vi "Car Wash Controller.vi"(8 "error in (no error)":errorcluster, 9 "Module Routes":refnum<user-event>[](array[refnum]), 11 "Event Registration Refnum":refnum<event-registration>) -> (0 "error out":errorcluster)   [LabVIEW 2016]
doc: "Car wash controller main"
uses:
  Architecture/Message Queue/Message Cluster.ctl
  Controls/Controller Status.ctl
  Simulated Console/Controls/Button state.ctl
  Controls/Steps.ctl
  Controls/Stations.ctl
  Controls/Waiting States.ctl
  Architecture/Modules.ctl
  Simulated Console/Controls/Entry Display.ctl
  Architecture/Message Queue/Message Queue.lvlib
panel:
  in  "debug":bool
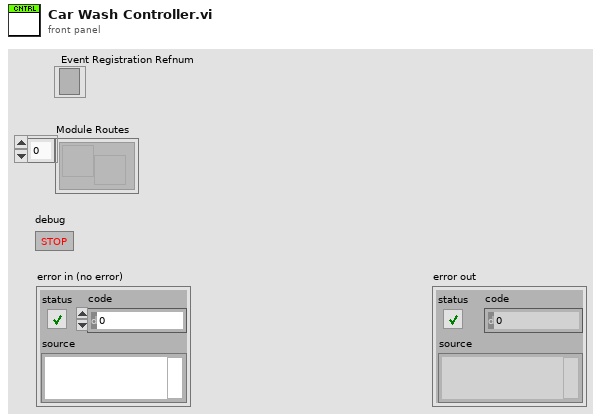
[diagram p1: front panel]
types:
  T1 = typedef "Controller Status.ctl" = cluster{"Module Routes":refnum<user-event>[], "Button States":T2[], "Current State":T3, "In Progress?":bool, "Out of Position?":bool, "Time Remaining":dbl, "Current Station":T4, "Waiting States":T5, "Chosen Cycles":cluster{"Under Body Wash":bool, "Bug Remover":bool, "Pre-Soak":bool, "High Pressure Wash (default)":bool, "Low Pressure Wax":bool, "Spot Free Rinse":bool, "Tire Shine Foam":bool, "Air Dry":bool}}
  T2 = typedef "Button state.ctl" = cluster{"Disabled State":enum8{"Enabled", "Disabled", "Disabled and Grayed Out"}, "State":bool}
  T3 = typedef "Steps.ctl" = enum16{"Under Body Wash", "Bug Remover", "Pre-Soak", "High Pressure Wash", "Low Pressure Wax", "Spot Free Rinse", "Tire Shine Foam", "Air Dry"}
  T4 = typedef "Stations.ctl" = enum16{"Entry", "Station 1", "Station 2", "Station 3", "Exit"}
  T5 = typedef "Waiting States.ctl" = enum16{"None", "for Start", "for Vehicle Position"}
  T6 = typedef "Entry Display.ctl" = cluster{"Text":string, "Color":u32}
  T7 = typedef "Modules.ctl" = enum16{"Database", "Car Wash Controller", "Console"}
  T8 = typedef "Error Severity.ctl" = enum16{"System Error", "Wash Error", "Minor"}
  T9 = cluster{"Under Body Wash":bool, "Bug Remover":bool, "Pre-Soak":bool, "High Pressure Wash (default)":bool, "Low Pressure Wax":bool, "Spot Free Rinse":bool, "Tire Shine Foam":bool, "Air Dry":bool}
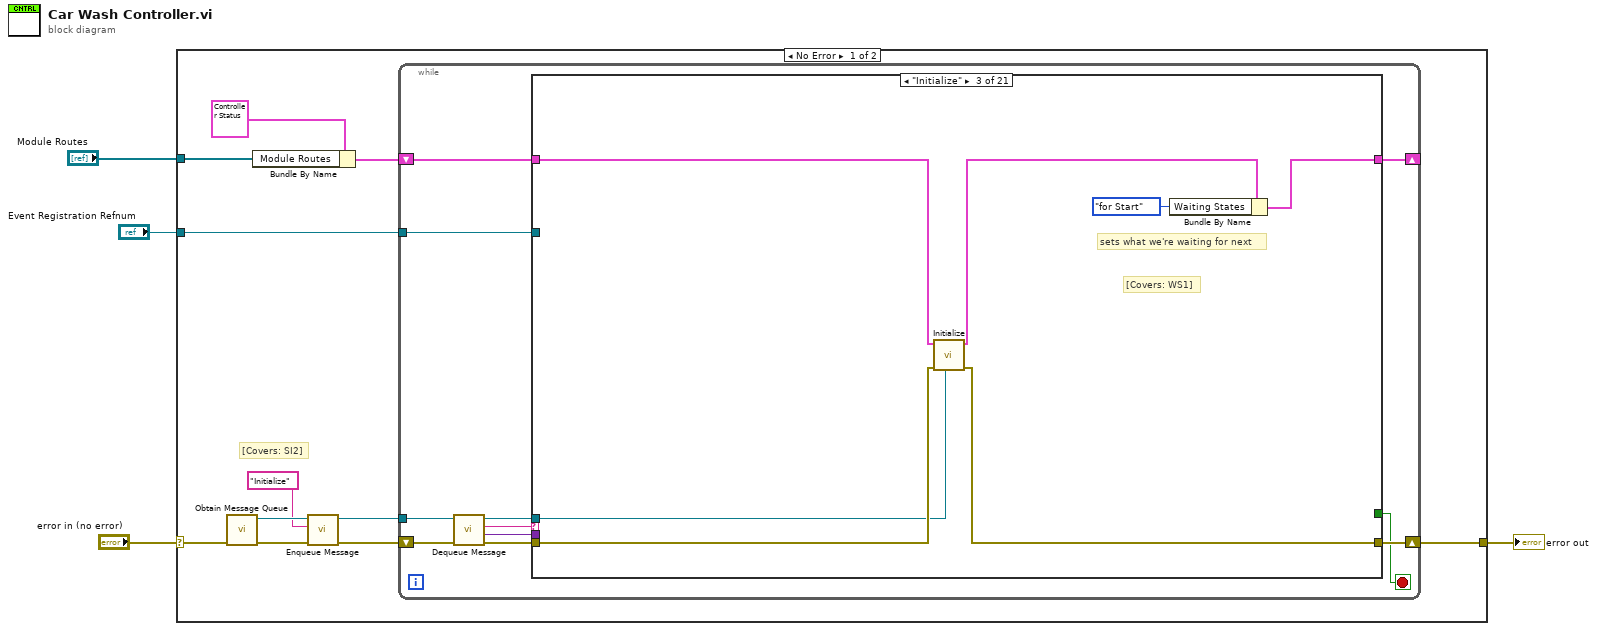
[diagram p0: block diagram]
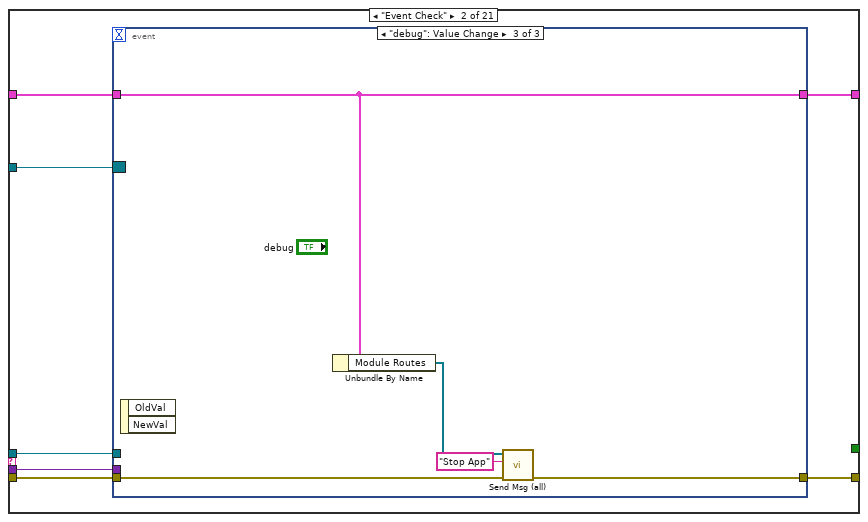
[diagram p3: hidden frame]
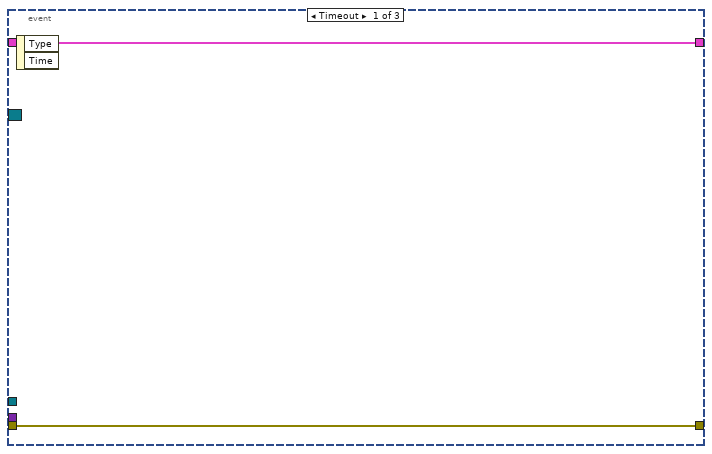
[diagram p4: hidden frame]
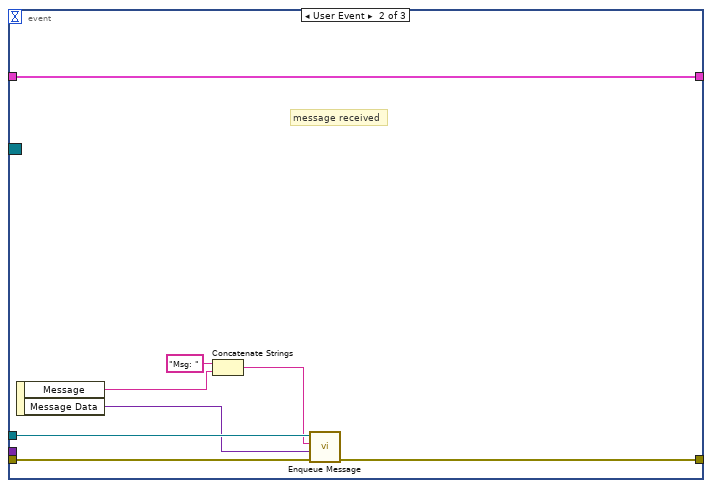
[diagram p5: hidden frame]
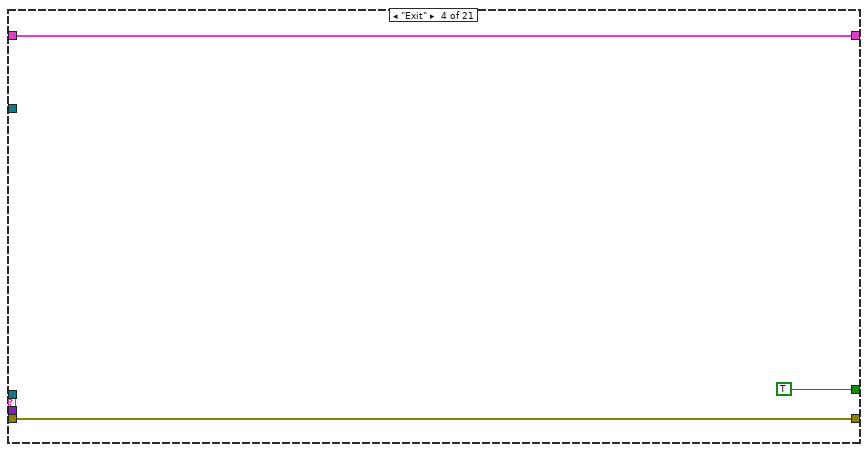
[diagram p6: hidden frame]
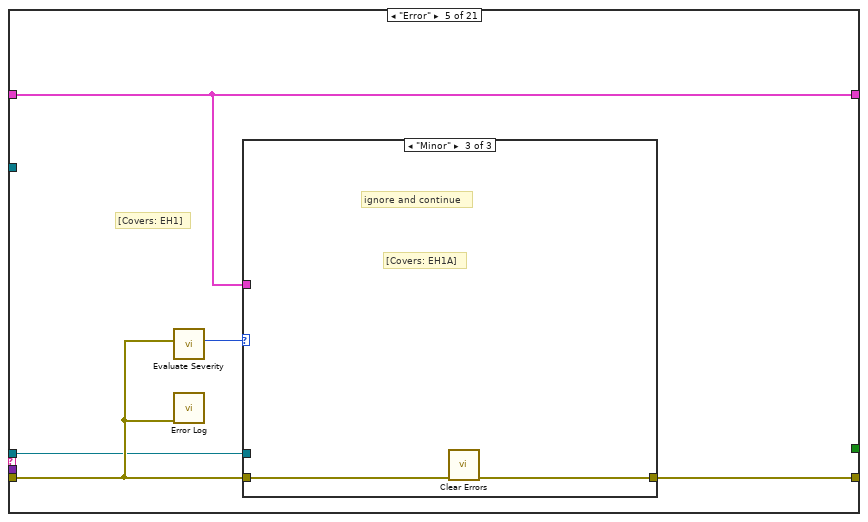
[diagram p7: hidden frame]
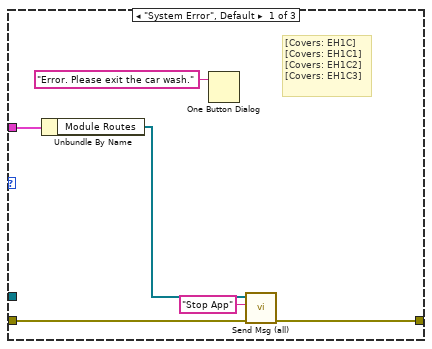
[diagram p8: hidden frame]
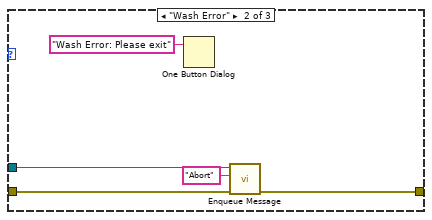
[diagram p9: hidden frame]
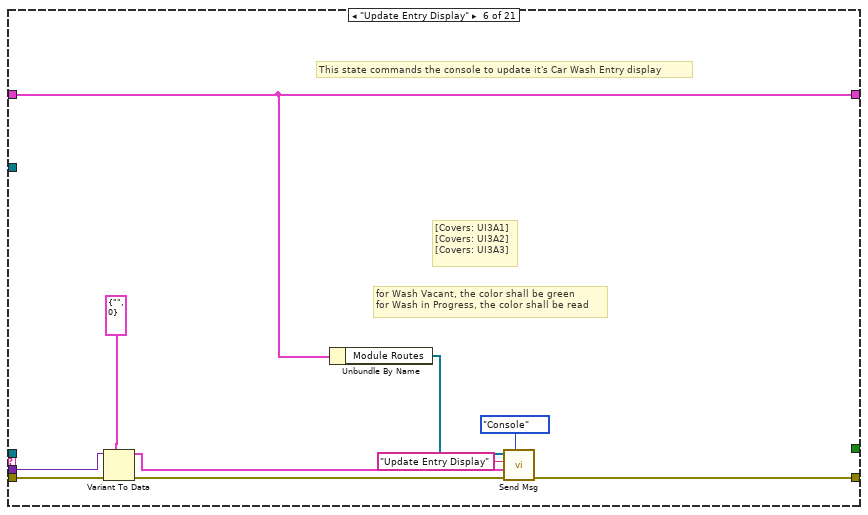
[diagram p10: hidden frame]
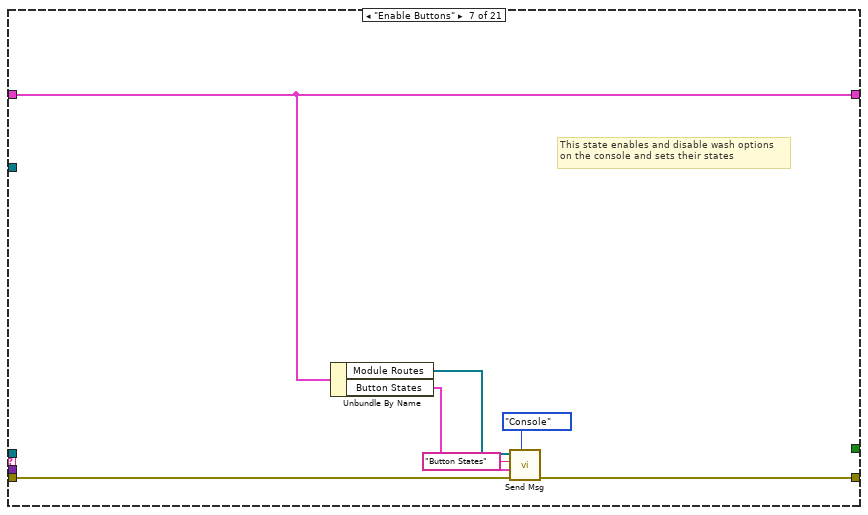
[diagram p11: hidden frame]
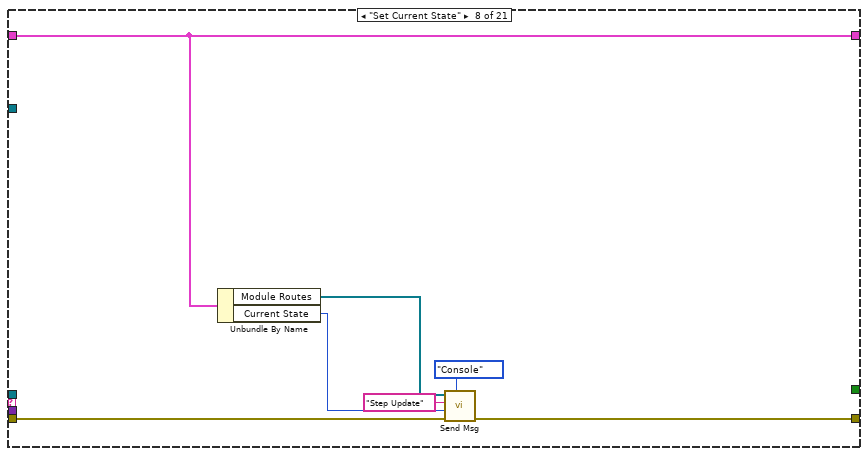
[diagram p12: hidden frame]
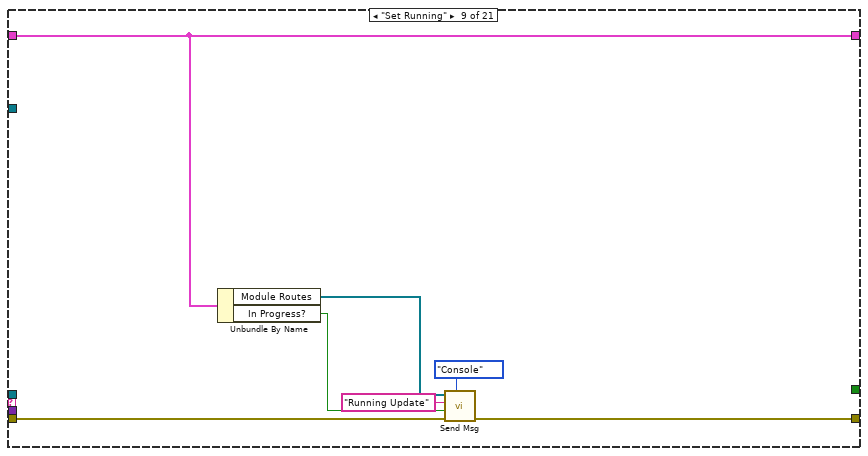
[diagram p13: hidden frame]
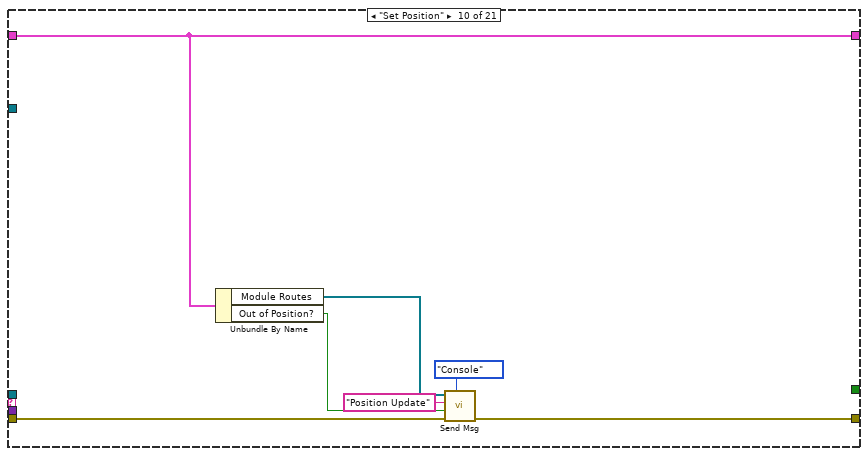
[diagram p14: hidden frame]
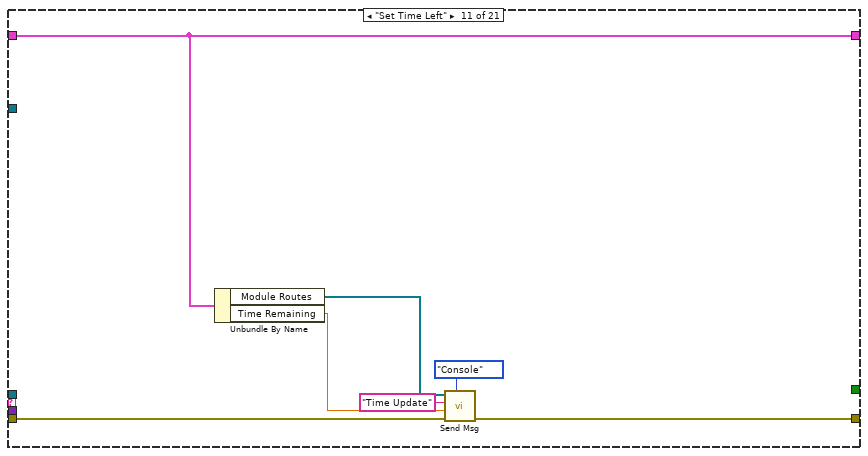
[diagram p15: hidden frame]
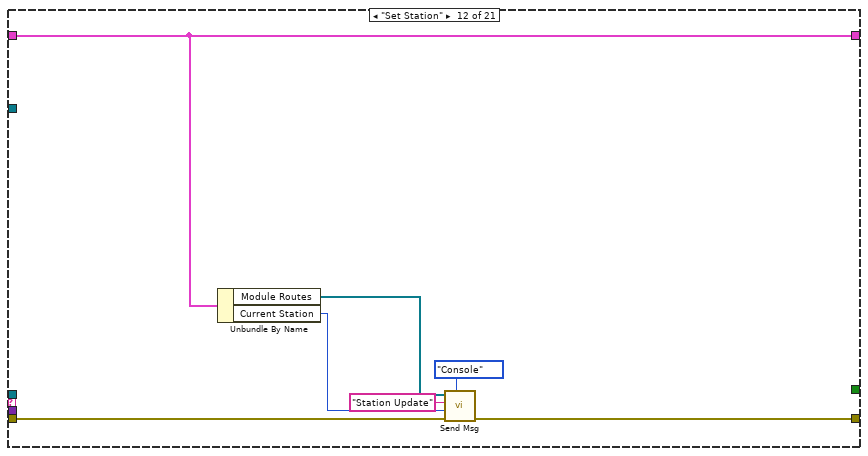
[diagram p16: hidden frame]
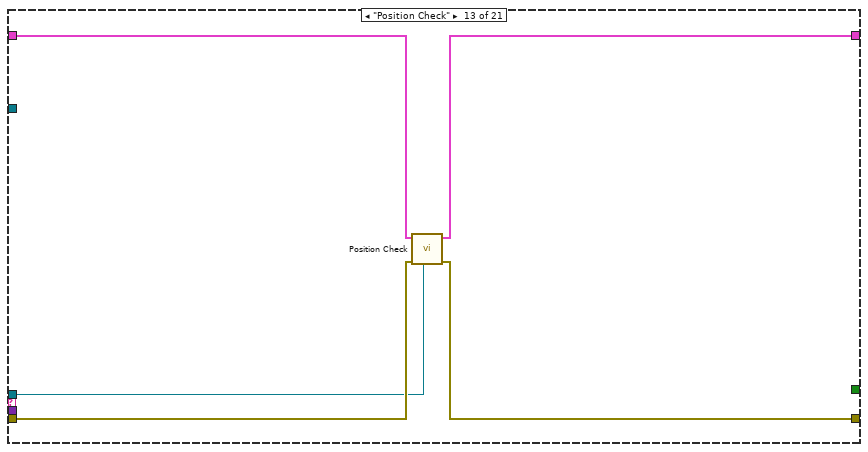
[diagram p17: hidden frame]
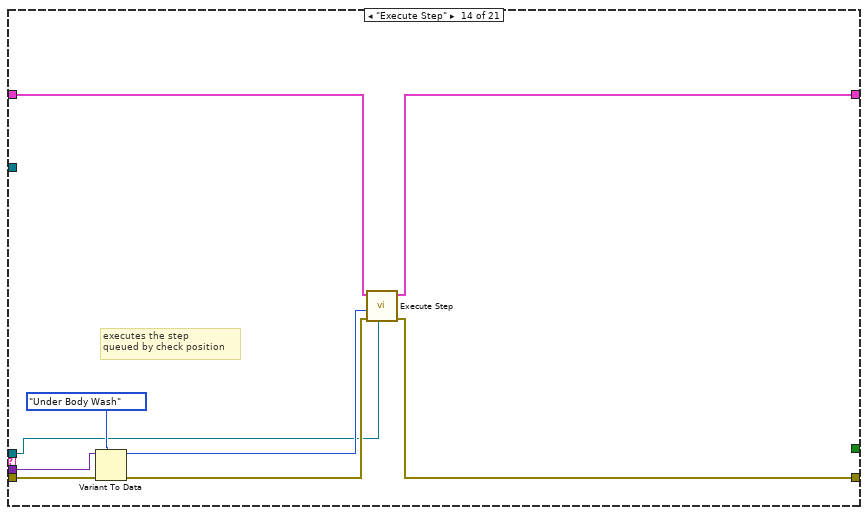
[diagram p18: hidden frame]
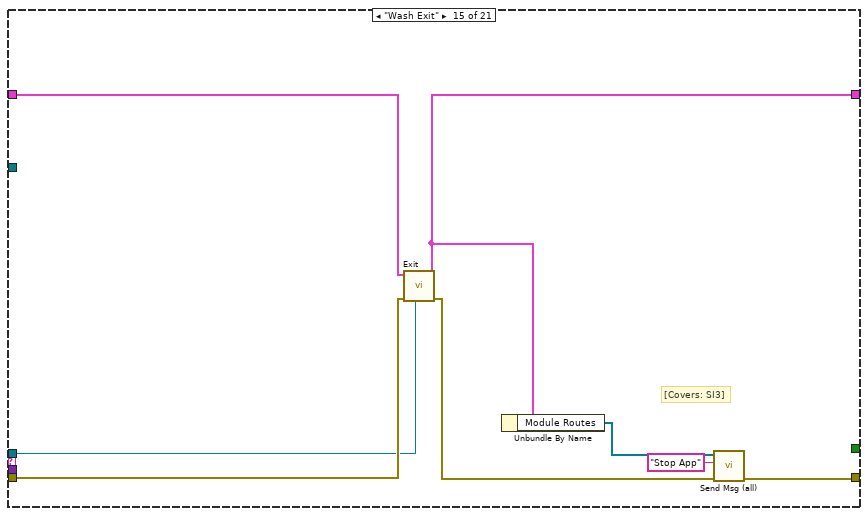
[diagram p19: hidden frame]
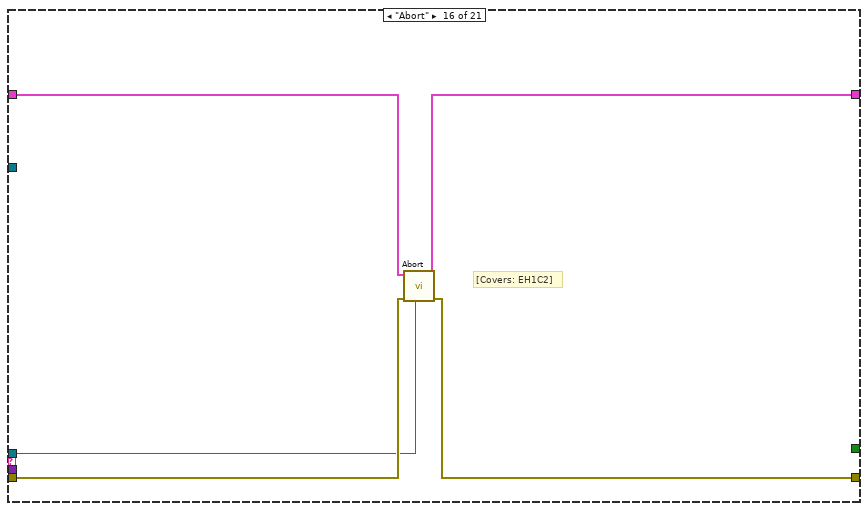
[diagram p20: hidden frame]
diagram:
  n1 = case shown="No Error" "error in (no error)" {
    selector: "error in (no error)" -> [w12 w198]
    tunnel: "Module Routes" -> [w14 _]
    tunnel: "Event Registration Refnum" -> [w13 _]
    tunnel: [w6 w198] -> w1
    frame No Error {
      # "[Covers: SI2]"
      n2 = call "Obtain Message Queue.vi"("error in (no error)"=w12) -> ("error out"=w11:errorcluster, "Message Queue"=w10:refnum<queue>)  [unwired: 9 in]
      n3 = Bundle By Name(cluster=T1 {"Module Routes"=[], "Button States"=[], "Current State"=enum."Under Body Wash", "In Progress?"=FALSE, "Out of Position?"=FALSE, "Time Remaining"=0.0, "Current Station"=enum."Entry", "Waiting States"=enum."None", "Chosen Cycles"={"Under Body Wash"=FALSE, "Bug Remover"=FALSE, "Pre-Soak"=FALSE, "High Pressure Wash (default)"=FALSE, "Low Pressure Wax"=FALSE, "Spot Free Rinse"=FALSE, "Tire Shine Foam"=FALSE, "Air Dry"=FALSE}} ("Status"), "Module Routes"=w14) -> (w5:T1)
      n4 = call "Enqueue Message.vi"("error in (no error)"=w11, "Message"="Initialize", "Message Queue"=w10) -> ("error out"=w8:errorcluster, "dup Message Queue"=w7:refnum<queue>)  [unwired: 7 in]
      n5 = while {
        tunnel: w13 -> [w26]
        shift-right: [w22] -> w6
        shift-left: w8 -> [w25]
        tunnel: w7 -> [w24]
        shift-right: [w16] -> _
        shift-left: w5 -> [w17]
        stop <- w18 stop-if-true
        n6 = call "Dequeue Message.vi"("error in (no error)"=w25, "Message Queue"=w24) -> ("error out"=w23:errorcluster, "Message Data"=w20:variant, "Message"=w19:string, "dup Message Queue"=w21:refnum<queue>)  [unwired: 6 in]
        n7 = case shown="\"Initialize\"" w19 {
          tunnel: w26 -> [_ w35 _ _ _ _ _ _ _ _ _ _ _ _ _ _ _ _ _ _ _]
          tunnel: w23 -> [w28 w34 w57 w60 w62 w84 w95 w102 w109 w116 w123 w130 w135 w144 w152 w157 w159 w164 w180 w189 w197]
          tunnel: [w28 w33 w56 w60 w64 w88 w94 w101 w108 w115 w122 w129 w134 w136 w148 w156 w159 w166 w170 w183 w195] -> w22
          tunnel: w21 -> [_ w32 w54 _ w61 _ _ _ _ _ _ _ w133 w139 w150 w153 _ w163 w169 w182 w196]
          tunnel: w20 -> [_ w31 _ _ _ w81 _ _ _ _ _ _ _ w143 _ _ _ _ w177 w187 _]
          tunnel: [_ _ _ TRUE _ _ _ _ _ _ _ _ _ _ _ _ _ _ _ _ _] -> w18
          tunnel: w17 -> [w27 w30 w55 w58 w63 w87 w93 w100 w107 w114 w121 w128 w132 w138 w151 w155 w158 w167 w176 w186 w192]
          tunnel: [w27 w29 w52 w58 w63 w87 w93 w100 w107 w114 w121 w128 w131 w137 w147 w154 w158 w167 w173 w186 w191] -> w16
          frame Default {
            # "invalid case"
          }
          frame "Event Check" {
            n8 = event shown="[2] \"debug\": Value Change" {
              selector: w35 -> [_ _ _]
              dyn-events: _ -> [_ _ _]
              timeout: _ -> [_ _ _]
              tunnel: [w37 w42 w49] -> w33
              tunnel: w34 -> [w37 w43 w50]
              tunnel: w32 -> [_ w41 _]
              tunnel: w31 -> [_ _ _]
              tunnel: w30 -> [w36 w38 w48]
              tunnel: [w36 w38 w48] -> w29
              event Timeout {
                n9 = event-data() -> ()  [unwired: 1 in, 2 out]
              }
              event User Event {
                # "message received"
                n10 = event-data() -> ("Message"=w44:string, "Message Data"=w40:variant)  [unwired: 1 in]
                n11 = Concatenate Strings("Msg: " ("string"), w44) -> (w39:string)
                n12 = call "Enqueue Message.vi"("error in (no error)"=w43, "Message Data"=w40, "Message"=w39, "Message Queue"=w41) -> ("error out"=w42:errorcluster)  [unwired: 6 in, 1 out]
              }
              event "debug": Value Change {
                n13 = event-data() -> ()  [unwired: 1 in, 2 out]
                n14 = Unbundle By Name(w48) -> ("Module Routes"=w47:refnum<user-event>[])
                n15 = call "Send Msg (all).vi"("error in (no error)"=w50, "Message"="Stop App", "Module Routes"=w47) -> ("error out"=w49:errorcluster)  [unwired: 8 in]
              }
            }
          }
          frame "Initialize" {
            # "[Covers: WS1]"
            # "sets what we're waiting for next"
            n16 = call "Initialize.vi"("Message Queue"=w54, "error in (no error)"=w57, "Status"=w55) -> ("error out"=w56:errorcluster, "Status"=w53:T1)  [unwired: 7 in]
            n17 = Bundle By Name(cluster=w53, "Waiting States"=Waiting_States."for Start") -> (w52:T1)
          }
          frame "Exit" {
          }
          frame "Error" {
            # "[Covers: EH1]"
            n18 = call "Evaluate Severity.vi"("error in (no error)"=w62) -> ("Severity"=w65:T8)  [unwired: 10 in]
            n19 = call "Error Log.vi"("error in (no error)"=w62) -> ()  [unwired: 11 in]
            n20 = case shown="\"Minor\"" w65 {
              tunnel: w62 -> [w70 w75 w78]
              tunnel: [w69 w74 w77] -> w64
              tunnel: w63 -> [w68 _ _]
              tunnel: w61 -> [_ w73 _]
              frame "System Error", Default {
                # "[Covers: EH1C]\n[Covers: EH1C1]\n[Covers: EH1C2]\n[Covers: EH1C3]"
                n21 = Unbundle By Name(w68) -> ("Module Routes"=w67:refnum<user-event>[])
                n22 = One Button Dialog(message="Error. Please exit the car wash.") -> ()  [unwired: 1 in, 1 out]
                n23 = call "Send Msg (all).vi"("error in (no error)"=w70, "Message"="Stop App", "Module Routes"=w67) -> ("error out"=w69:errorcluster)  [unwired: 8 in]
              }
              frame "Wash Error" {
                n24 = One Button Dialog(message="Wash Error: Please exit") -> ()  [unwired: 1 in, 1 out]
                n25 = call "Enqueue Message.vi"("error in (no error)"=w75, "Message"="Abort", "Message Queue"=w73) -> ("error out"=w74:errorcluster)  [unwired: 7 in, 1 out]
              }
              frame "Minor" {
                # "[Covers: EH1A]"
                # "ignore and continue"
                n26 = call <vilib>:"Clear Errors.vi"("error in (no error)"=w78) -> ("error out"=w77:errorcluster)  [unwired: 5 in, 1 out]
              }
            }
          }
          frame "Update Entry Display" {
            # "for Wash Vacant, the color shall be green\nfor Wash in Progress, the color shall be read"
            # "[Covers: UI3A1]\n[Covers: UI3A2]\n[Covers: UI3A3]"
            # "This state commands the console to update it's Car Wash Entry display"
            n27 = Variant To Data(error in=w84, type=T6 {"Text"="", "Color"=0}, Variant=w81) -> (data=w80:T6, error out=w83:errorcluster)
            n28 = Unbundle By Name(w87) -> ("Module Routes"=w86:refnum<user-event>[])
            n29 = call "Send Msg.vi"("Module"=Modules."Console", "error in (no error)"=w83, "Message Data"=w80, "Message"="Update Entry Display", "Module Routes"=w86) -> ("error out"=w88:errorcluster)  [unwired: 6 in]
          }
          frame "Enable Buttons" {
            # "This state enables and disable wash options\non the console and sets their states"
            n30 = Unbundle By Name(w93) -> ("Module Routes"=w92:refnum<user-event>[], "Button States"=w91:T2[])
            n31 = call "Send Msg.vi"("Module"=Modules."Console", "error in (no error)"=w95, "Message Data"=w91, "Message"="Button States", "Module Routes"=w92) -> ("error out"=w94:errorcluster)  [unwired: 6 in]
          }
          frame "Set Current State" {
            n32 = Unbundle By Name(w100) -> ("Module Routes"=w99:refnum<user-event>[], "Current State"=w97:T3)
            n33 = call "Send Msg.vi"("Module"=Modules."Console", "error in (no error)"=w102, "Message Data"=w97, "Message"="Step Update", "Module Routes"=w99) -> ("error out"=w101:errorcluster)  [unwired: 6 in]
          }
          frame "Set Running" {
            n34 = Unbundle By Name(w107) -> ("Module Routes"=w106:refnum<user-event>[], "In Progress?"=w104:bool)
            n35 = call "Send Msg.vi"("Module"=Modules."Console", "error in (no error)"=w109, "Message Data"=w104, "Message"="Running Update", "Module Routes"=w106) -> ("error out"=w108:errorcluster)  [unwired: 6 in]
          }
          frame "Set Position" {
            n36 = Unbundle By Name(w114) -> ("Module Routes"=w113:refnum<user-event>[], "Out of Position?"=w111:bool)
            n37 = call "Send Msg.vi"("Module"=Modules."Console", "error in (no error)"=w116, "Message Data"=w111, "Message"="Position Update", "Module Routes"=w113) -> ("error out"=w115:errorcluster)  [unwired: 6 in]
          }
          frame "Set Time Left" {
            n38 = Unbundle By Name(w121) -> ("Module Routes"=w120:refnum<user-event>[], "Time Remaining"=w118:dbl)
            n39 = call "Send Msg.vi"("Module"=Modules."Console", "error in (no error)"=w123, "Message Data"=w118, "Message"="Time Update", "Module Routes"=w120) -> ("error out"=w122:errorcluster)  [unwired: 6 in]
          }
          frame "Set Station" {
            n40 = Unbundle By Name(w128) -> ("Module Routes"=w127:refnum<user-event>[], "Current Station"=w125:T4)
            n41 = call "Send Msg.vi"("Module"=Modules."Console", "error in (no error)"=w130, "Message Data"=w125, "Message"="Station Update", "Module Routes"=w127) -> ("error out"=w129:errorcluster)  [unwired: 6 in]
          }
          frame "Position Check" {
            n42 = call "Position Check.vi"("Message Queue"=w133, "error in (no error)"=w135, "Status"=w132) -> ("error out"=w134:errorcluster, "Status"=w131:T1)  [unwired: 7 in]
          }
          frame "Execute Step" {
            # "executes the step\nqueued by check position"
            n43 = Variant To Data(error in=w144, type=Steps."Under Body Wash" ("Current State"), Variant=w143) -> (data=w140:T3, error out=w141:errorcluster)
            n44 = call "Execute Step.vi"("Message Queue"=w139, "error in (no error)"=w141, "Step"=w140, "Status"=w138) -> ("error out"=w136:errorcluster, "Status"=w137:T1)  [unwired: 6 in]
          }
          frame "Wash Exit" {
            # "[Covers: SI3]"
            n45 = call "Exit.vi"("Message Queue"=w150, "error in (no error)"=w152, "Status"=w151) -> ("error out"=w149:errorcluster, "Status"=w147:T1)  [unwired: 7 in]
            n46 = Unbundle By Name(w147) -> ("Module Routes"=w146:refnum<user-event>[])
            n47 = call "Send Msg (all).vi"("error in (no error)"=w149, "Message"="Stop App", "Module Routes"=w146) -> ("error out"=w148:errorcluster)  [unwired: 8 in]
          }
          frame "Abort" {
            # "[Covers: EH1C2]"
            n48 = call "Abort.vi"("Message Queue"=w153, "error in (no error)"=w157, "Status"=w155) -> ("error out"=w156:errorcluster, "Status"=w154:T1)  [unwired: 7 in]
          }
          frame "=== Messages ===" {
            # "placeholder"
          }
          frame "Msg: Stop App" {
            # "[Covers: EH1C1]\n[Covers: EH1C2]\n[Covers: EH1C3]"
            n49 = call "Enqueue Message.vi"("error in (no error)"=w164, "Message"="Abort", "Message Queue"=w163) -> ("error out"=w162:errorcluster, "dup Message Queue"=w161:refnum<queue>)  [unwired: 7 in]
            n50 = call "Enqueue Message.vi"("error in (no error)"=w162, "Message"="Exit", "Message Queue"=w161) -> ("error out"=w166:errorcluster)  [unwired: 7 in, 1 out]
          }
          frame "Msg: Start Wash" {
            n51 = Unbundle By Name(w176) -> ("Chosen Cycles"=w179:T9)
            n52 = Variant To Data(error in=w180, type=w179, Variant=w177) -> (data=w178:T9, error out=w175:errorcluster)
            n53 = Bundle By Name(cluster=w176, "Chosen Cycles"=w178) -> ()  [unwired: 1 out]
            n54 = call "Start.vi"("Message Queue"=w169, "error in (no error)"=w175, "Status"=w176) -> ("error out"=w171:errorcluster, "Status"=w174:T1)  [unwired: 7 in]
            n55 = Bundle By Name(cluster=w174, "Waiting States"=Waiting_States."for Vehicle Position") -> (w173:T1)
            n56 = call "Enqueue Message.vi"("error in (no error)"=w171, "Message"="Position Check", "Message Queue"=w169) -> ("error out"=w170:errorcluster)  [unwired: 7 in, 1 out]
          }
          frame "Msg: Vehicle Position Update" {
            # "[Covers: VS1]\n[Covers: VS2]\n[Covers: VS3]\n[Covers: VS4]"
            # "Check to see whether we are now in the right\nposition or moved into a wrong position"
            n57 = Unbundle By Name(w186) -> ("Current Station"=w188:T4)
            n58 = Variant To Data(error in=w189, type=w188, Variant=w187) -> (data=w185:T4, error out=w184:errorcluster)
            n59 = Bundle By Name(cluster=w186, "Current Station"=w185) -> ()  [unwired: 1 out]
            n60 = call "Enqueue Message.vi"("error in (no error)"=w184, "Message"="Position Check", "Message Queue"=w182) -> ("error out"=w183:errorcluster)  [unwired: 7 in, 1 out]
          }
          frame "Msg: Wash Error" {
            # "[Covers: EH1B1]\n[Covers: EH1B2]"
            n61 = One Button Dialog(message="Wash Error. Please Exit") -> ()  [unwired: 1 in, 1 out]
            n62 = call "Enqueue Message.vi"("error in (no error)"=w197, "Message"="Abort", "Message Queue"=w196) -> ("error out"=w195:errorcluster)  [unwired: 7 in, 1 out]
            n63 = Bundle By Name(cluster=w192, "Waiting States"=Waiting_States."for Vehicle Position") -> (w191:T1)
          }
        }
      }
    }
    frame Error {
    }
  }
  "error out" <- w1
